vi "ConvertSweepToWfm.vi"(10 "sweep":cluster{"frequency":dbl, "amplitude":dbl}[](array[cluster])) -> (2 "array":sgl[](array[numeric]))   [LabVIEW 2017, in "EmsaDataEventCreator.lvlib"]
uses:
  <vilib>/addons/InsightCM/Devices/Shared/Emsa/EmsaDataEventCreator/EmsaDataEventCreator.lvlib
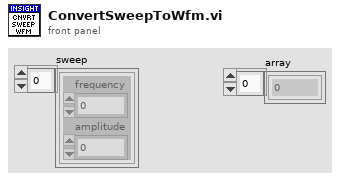
[diagram p1: front panel]
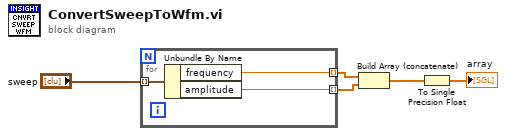
[diagram p0: block diagram]
diagram:
  n1 = for {
    tunnel: "sweep" -> [w8] mode=indexing
    tunnel: [w7] -> w3 mode=indexing
    tunnel: [w6] -> w2 mode=indexing
    n2 = Unbundle By Name(w8) -> ("frequency"=w7:dbl, "amplitude"=w6:dbl)
  }
  n3 = Build Array (concatenate)(w3, w2) -> (w1:dbl[])
  n4 = To Single Precision Float(number=w1) -> (single precision float=→"array":sgl[])
